vi "Run.vi"(8 "error in (no error)":errorcluster, 11 "socket REP in":refnum<class "socket REP.lvclass">) -> (0 "error out":errorcluster, 3 "socket REP out":refnum<class "socket REP.lvclass">)   [LabVIEW 2018, in "socket REP.lvclass"]
uses:
  socket REP.lvclass
  C:/Users/devstaff/sparc4/s4gui/Versao ZeroMQ REQ-REP/SPARC4_GUI -v1.0.8 - com pacote communication manager/communication-manager/Socket/Socket.lvclass
  Socket/Socket.lvclass
  State Machine/CM_State Machine.lvclass
  RxTx/CM_RxTx.lvclass
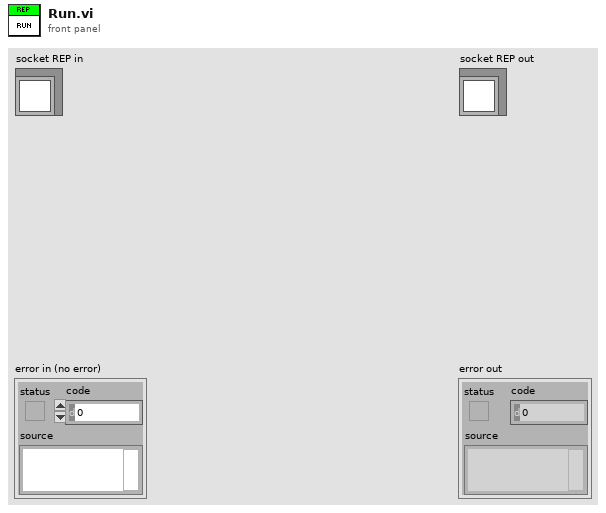
[diagram p1: front panel]
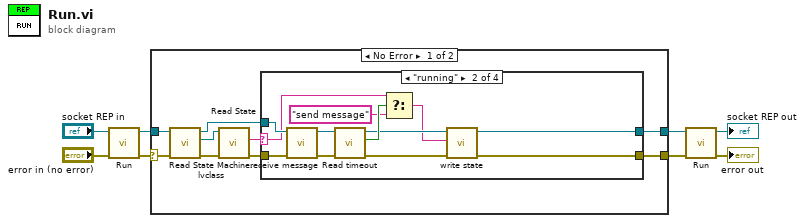
[diagram p0: block diagram]
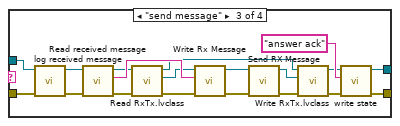
[diagram p3: hidden frame]
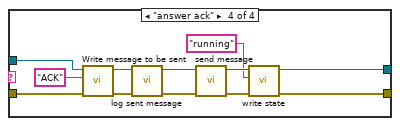
[diagram p4: hidden frame]
diagram:
  n1 = call-parent "Run.vi"("error in (no error)"="error in (no error)", "Socket in"="socket REP in") -> ("error out"=w5:errorcluster, "Socket out"=w6:refnum<class "socket REP.lvclass">)  [unwired: 8 in]
  n2 = case shown="No Error" w5 {
    selector: w5 -> [w11 w63]
    tunnel: w6 -> [w12 w64]
    tunnel: [w15 w64] -> w4
    tunnel: [w16 w63] -> w3
    frame No Error {
      n3 = call-dynamic "Read State Machine.lvclass.vi"("error in (no error)"=w11, "Socket in"=w12) -> ("error out"=w10:errorcluster, "State Machine.lvclass"=w13:refnum<class "CM_State Machine.lvclass">, "Socket out"=w9:refnum<class "socket REP.lvclass">)  [unwired: 7 in]
      n4 = call-dynamic "Read State.vi"("error in (no error)"=w10, "State Machine in"=w13) -> ("error out"=w14:errorcluster, "State"=w17:string)  [unwired: 7 in, 1 out]
      n5 = case shown="\"running\"" w17 {
        selector: w17 -> [_ w20 _ _]
        tunnel: [w18 w24 w42 w59] -> w15
        tunnel: [w19 w23 w41 w58] -> w16
        tunnel: w14 -> [w19 w30 w35 w55]
        tunnel: w9 -> [w18 w31 w32 w61]
        frame Default {
        }
        frame "running" {
          n6 = call-dynamic "receive message.vi"("error in (no error)"=w30, "Socket in"=w31) -> ("error out"=w28:errorcluster, "Socket out"=w29:refnum<class "socket REP.lvclass">)  [unwired: 8 in]
          n7 = call-dynamic "Read timeout.vi"("error in (no error)"=w28, "Socket in"=w29) -> ("error out"=w22:errorcluster, "timeout"=w27:bool, "Socket out"=w25:refnum<class "socket REP.lvclass">)  [unwired: 7 in]
          n8 = Select(t=w20, s=w27, f="send message") -> (s? t:f=w21:string)
          n9 = call "write state.vi"("error in (no error)"=w22, "State"=w21, "Socket in"=w25) -> ("error out"=w23:errorcluster, "Socket out"=w24:refnum<class "socket REP.lvclass">)  [unwired: 7 in]
        }
        frame "send message" {
          n10 = call "log received message.vi"("error in (no error)"=w35, "Socket in"=w32) -> ("error out"=w34:errorcluster, "Socket out"=w33:refnum<class "socket REP.lvclass">)  [unwired: 8 in]
          n11 = call-dynamic "Read received message.vi"("error in (no error)"=w34, "Socket in"=w33) -> ("error out"=w39:errorcluster, "received message"=w49:string, "Socket out"=w46:refnum<class "socket REP.lvclass">)  [unwired: 7 in]
          n12 = call-dynamic "Read RxTx.lvclass.vi"("error in (no error)"=w39, "Socket in"=w46) -> ("error out"=w38:errorcluster, "RxTx.lvclass"=w47:refnum<class "CM_RxTx.lvclass">, "Socket out"=w44:refnum<class "socket REP.lvclass">)  [unwired: 7 in]
          n13 = call "Write Rx Message.vi"("error in (no error)"=w38, "Rx Message"=w49, "RxTx in"=w47) -> ("error out"=w48:errorcluster, "RxTx out"=w50:refnum<class "CM_RxTx.lvclass">)  [unwired: 7 in]
          n14 = call "Send RX Message.vi"("error in (no error)"=w48, "RxTx in"=w50) -> ("error out"=w43:errorcluster, "RxTx out"=w45:refnum<class "CM_RxTx.lvclass">)  [unwired: 8 in]
          n15 = call-dynamic "Write RxTx.lvclass.vi"("error in (no error)"=w43, "RxTx.lvclass"=w45, "Socket in"=w44) -> ("error out"=w36:errorcluster, "Socket out"=w37:refnum<class "socket REP.lvclass">)  [unwired: 7 in]
          n16 = call "write state.vi"("error in (no error)"=w36, "State"="answer ack", "Socket in"=w37) -> ("error out"=w41:errorcluster, "Socket out"=w42:refnum<class "socket REP.lvclass">)  [unwired: 7 in]
        }
        frame "answer ack" {
          n17 = call-dynamic "Write message to be sent.vi"("error in (no error)"=w55, "message to be sent"="ACK", "Socket in"=w61) -> ("error out"=w51:errorcluster, "Socket out"=w54:refnum<class "socket REP.lvclass">)  [unwired: 7 in]
          n18 = call "log sent message.vi"("error in (no error)"=w51, "Socket in"=w54) -> ("error out"=w52:errorcluster, "Socket out"=w53:refnum<class "socket REP.lvclass">)  [unwired: 8 in]
          n19 = call "send message.vi"("error in (no error)"=w52, "Socket in"=w53) -> ("error out"=w57:errorcluster, "Socket out"=w60:refnum<class "socket REP.lvclass">)  [unwired: 8 in]
          n20 = call "write state.vi"("error in (no error)"=w57, "State"="running", "Socket in"=w60) -> ("error out"=w58:errorcluster, "Socket out"=w59:refnum<class "socket REP.lvclass">)  [unwired: 7 in]
        }
      }
    }
    frame Error {
    }
  }
  n21 = call-parent "Run.vi"("error in (no error)"=w3, "Socket in"=w4) -> ("error out"=→"error out":errorcluster, "Socket out"=→"socket REP out":refnum<class "socket REP.lvclass">)  [unwired: 8 in]
